vi "Trim Quotes.vi"(11 "String":string) -> (2 "Quotes Trimmed":bool, 3 "String without Quotes":string)   [LabVIEW 2015, in "NI_Azure_JSON Parsing.lvlib"]
uses:
  NI_Azure_JSON Parsing.lvlib
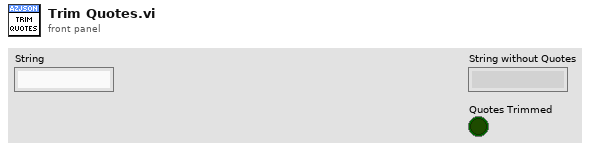
[diagram p1: front panel]
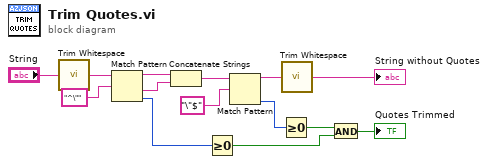
[diagram p0: block diagram]
diagram:
  n1 = call <vilib>:"Trim Whitespace.vi"("string"="String") -> ("trimmed string"=w8:string)  [unwired: 1 in]
  n2 = Match Pattern(string=w8, regular expression="^\"") -> (before substring=w10:string, after substring=w11:string, offset past match=w5:i32)  [unwired: 1 in, 1 out]
  n3 = Concatenate Strings(w10, w11) -> (w12:string)
  n4 = Greater Or Equal To 0?(x=w5) -> (x >= 0?=w2:bool)
  n5 = Match Pattern(string=w12, regular expression="\"$") -> (before substring=w14:string, offset past match=w4:i32)  [unwired: 1 in, 2 out]
  n6 = Greater Or Equal To 0?(x=w4) -> (x >= 0?=w3:bool)
  n7 = call <vilib>:"Trim Whitespace.vi"("string"=w14) -> ("trimmed string"=→"String without Quotes":string)  [unwired: 1 in]
  n8 = And(x=w3, y=w2) -> (x .and. y?=→"Quotes Trimmed":bool)
